vi "USRP_generator.vi"(4 "Y":cdb[][](array[numeric]), 9 "input cluster":T2={"USRP name"="B200", "active antenna"="TX1", "Freq"=1575450000.0, "Doppler"=0.0, " IQ rate(дискретизацтя)"=4092000.0, " Gain(dB)"=-10.0}) -> (0 "error out":errorcluster)   [LabVIEW 2020]
uses:
  AppData/Local/Programs/Python/Python35-32/Control 1.ctl
  <extravilib>/ChannelInstances/High Speed Stream-c(dbl,dbl,a[.](cdb))/_Read For Replicate.vi
  <extravilib>/ChannelInstances/High Speed Stream-c(dbl,dbl,a[.](cdb))/Instantiate.vi
  <extravilib>/ChannelInstances/High Speed Stream-c(dbl,dbl,a[.](cdb))/)Channel.vi
  <extravilib>/ChannelInstances/High Speed Stream-c(dbl,dbl,a[.](cdb))/Abort Signal/Init Signal.vi
  <instrlib>/niUSRP/niUSRP Write Tx Data (CDB Cluster).vi
  <vilib>/measure/maspectr.llb/FFT Power Spectrum and PSD for 1 Chan (CDB).vi
  <extravilib>/ChannelInstances/High Speed Stream-c(dbl,dbl,a[.](cdb)).lvlib
  <vilib>/measure/NI_MAPro.lvlib
panel:
  in  "Boolean":bool
  out "relative seconds":dbl format="%_19f"
  out "error out 2":errorcluster
  out "Waveform Graph 2":cluster{"f0":dbl, "df":dbl, "magnitude":dbl[]}(graph)
  out "Waveform Graph":waveform(dbl)(graph)
  in  "stop":bool
  in  "Целое число строк записанного файла":i32=1000
  in  "Timeout":dbl=10.0
  out "coerced gain(dB":dbl
  out "coerced carrier frequency":dbl
  out "coerced IQ rate":dbl
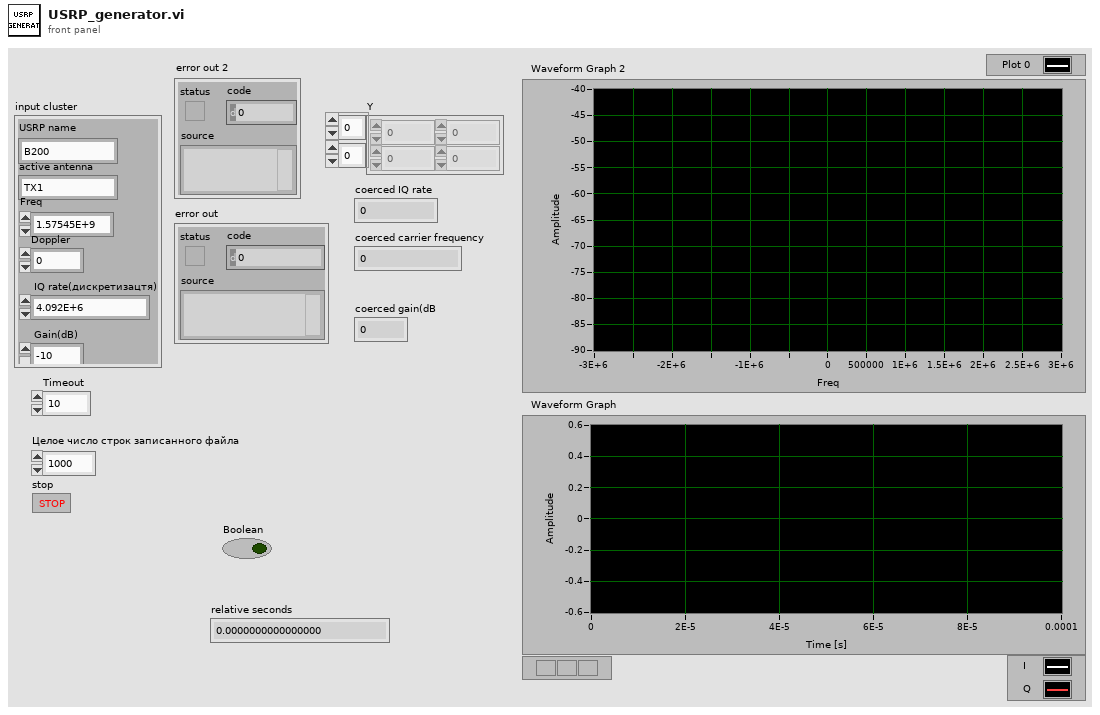
[diagram p1: front panel]
types:
  T1 = typedef "Control 1.ctl" = string
  T2 = cluster{"USRP name":T1, "active antenna":string, "Freq":dbl, "Doppler":dbl, " IQ rate(дискретизацтя)":dbl, " Gain(dB)":dbl}
  T3 = typedef "High Speed Stream-c(dbl,dbl,a[.](cdb)).lvlib/)Channel.ctl" = refnum<queue>
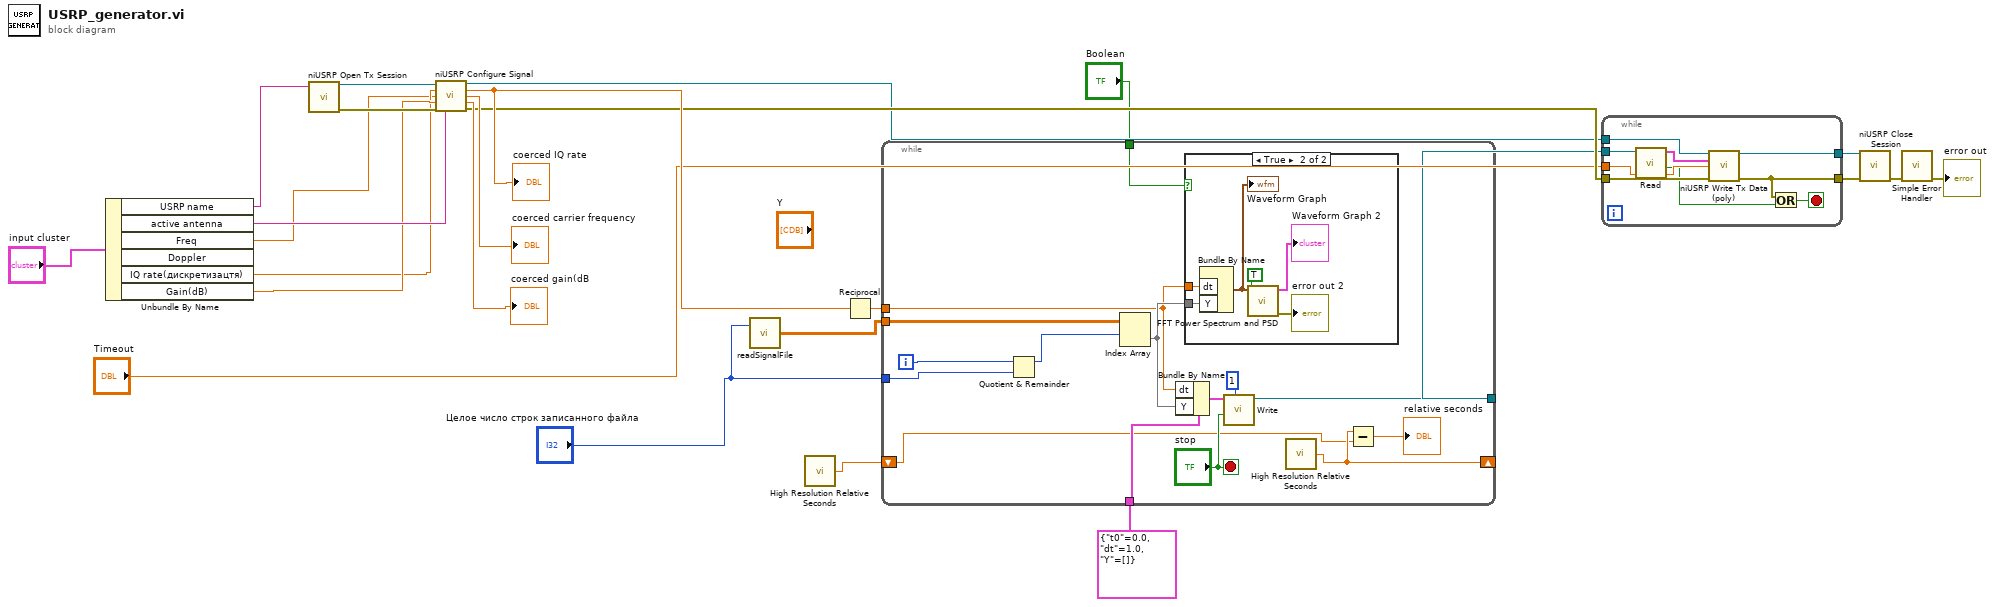
[diagram p0: block diagram]
diagram:
  n1 = Unbundle By Name("input cluster") -> ("USRP name"=w15:T1, "active antenna"=w14:string, "Freq"=w3:dbl, "IQ rate(дискретизацтя)"=w12:dbl, "Gain(dB)"=w13:dbl)  [unwired: 1 out]
  n2 = call <instrlib>:"niUSRP Open Tx Session.vi"("device names"=w15) -> ("session handle out"=w25:refnum<k15>, "error out"=w20:errorcluster)  [unwired: 13 in]
  n3 = call <instrlib>:"niUSRP Configure Signal.vi"("session handle"=w25, "IQ rate"=w12, "carrier frequency"=w3, "gain"=w13, "error in (no error)"=w20, "active antenna"=w14) -> ("session handle out"=w18:refnum<k15>, "coerced IQ rate"=w22:dbl, "coerced carrier frequency"=→"coerced carrier frequency":dbl, "coerced gain"=→"coerced gain(dB":dbl, "error out"=w19:errorcluster)  [unwired: 5 in]
  "coerced IQ rate" <- w22
  n4 = call "readSignalFile.vi"("Целое число строк записанного файла"="Целое число строк записанного файла") -> ("Array 2"=w5:cdb[][])  [unwired: 1 in]
  n5 = call <vilib>:"High Resolution Relative Seconds.vi"() -> ("relative seconds"=w1:dbl)
  n6 = Reciprocal(x=w22) -> (1/x=w7:dbl)
  n7 = while {
    tunnel: w5 -> [w40]
    tunnel: w7 -> [w34]
    tunnel: [w37] -> w6
    tunnel: cluster{"t0":dbl, "dt":dbl, "Y":cdb[]} {"t0"=0.0, "dt"=1.0, "Y"=[]} ("data") -> [w39]
    tunnel: "Целое число строк записанного файла" -> [w31]
    tunnel: "Boolean" -> [w29]
    shift-right: [w28] -> _
    shift-left: w1 -> [w27]
    i -> [w32]
    stop <- "stop" stop-if-true
    n8 = Quotient & Remainder(x=w32, y=w31) -> (x-y*floor(x/y)=w30:i32)  [unwired: 1 out]
    n9 = Index Array(array=w40, index (row)=w30) -> (element=w35:cdb[])  [unwired: 1 in]
    n10 = Bundle By Name(cluster=w39, "dt"=w34, "Y"=w35) -> (w38:cluster{"t0":dbl, "dt":dbl, "Y":cdb[]})
    n11 = case shown="True" w29 {
      tunnel: w35 -> [_ w45]
      tunnel: w34 -> [_ w44]
      frame False {
      }
      frame True {
        n12 = Bundle By Name("dt"=w44, "Y"=w45) -> (w43:waveform(cdb))  [unwired: 1 in]
        "Waveform Graph" <- w43
        n13 = call-poly <vilib>:"FFT Power Spectrum and PSD.vi"("dB On (F)"=TRUE, "time signal"=w43) -> ("error out"=→"error out 2":errorcluster, "Power Spectrum / PSD"=→"Waveform Graph 2":cluster{"f0":dbl, "df":dbl, "magnitude":dbl[]})  [unwired: 6 in, 2 out]
      }
    }
    n14 = call <extravilib>:"Write.vi"("size (unlimited)"=1, "last element? (F)"="stop", "element"=w38) -> ("channel"=w37:T3)  [unwired: 6 in, 2 out]
    n15 = call <vilib>:"High Resolution Relative Seconds.vi"() -> ("relative seconds"=w28:dbl)
    n16 = Subtract(x=w28, y=w27) -> (x-y=→"relative seconds":dbl)
  }
  n17 = while {
    tunnel: w18 -> [w51]
    tunnel: [w55] -> w17
    tunnel: [w53] -> w21
    tunnel: w19 -> [w54]
    tunnel: "Timeout" -> [w50]
    tunnel: w6 -> [w49]
    stop <- w52 stop-if-true
    n18 = call <extravilib>:"Read.vi"("channel"=w49) -> ("done?"=w48:bool, "element"=w47:cluster{"t0":dbl, "dt":dbl, "Y":cdb[]})  [unwired: 6 in, 3 out]
    n19 = call-poly <instrlib>:"niUSRP Write Tx Data (poly).vi"("session handle"=w51, "data"=w47, "timeout"=w50, "error in (no error)"=w54) -> ("session handle out"=w55:refnum<k15>, "error out"=w53:errorcluster)  [unwired: 10 in]
    n20 = Or(x=w53, y=w48) -> (x .or. y?=w52:bool)
  }
  n21 = call <instrlib>:"niUSRP Close Session.vi"("session handle"=w17, "error in (no error)"=w21) -> ("error out"=w10:errorcluster)  [unwired: 13 in]
  n22 = call <vilib>:"Simple Error Handler.vi"("error in (no error)"=w10) -> ("error out"=→"error out":errorcluster)  [unwired: 4 in, 4 out]
